vi "tkrsa6100 Config Spectrum Settings.vi"(0 "VISA Resource Name":refnum<visa-resource-name>, 1 "Set/Read\nSpectrum Setting (SET)":enum16{"SET", "READ"}(ring), 2 "Spectrum Settings\n (CENTER FREQUENCY)":T2(ring), 3 "Center Freq\n(MHz)(100)":dbl=100.0 min=0.0 max=20000.0 step=1e-06, 4 "Freq Span\n(MHz)(40)":dbl=40.0 min=1e-05 max=20000.0 step=1e-06, 5 "error in (no error)":errorcluster, 6 "Start Freq\n(MHz)(100)":dbl=100.0 min=0.0 max=14000.0 step=1e-06, 7 "Stop Freq\n(MHz)(1000)":dbl=1000.0 min=0.0 max=14000.0 step=1e-06, 8 "Freq Step\n(MHz)(10)":dbl=10.0 min=0.0 max=14000.0 step=1e-06, 9 "# Points\n(801)":enum16{"801", "2401", "4001", "8001", "10401"}(ring), 10 "Optimization\n(AUTO)":enum16{"AUTO", "DYNAMIC RANGE", "MIN NOISE"}(ring), 11 "Res BW (KHz)\n(300)":dbl=300.0 min=0.001 max=10000.0 step=0.001 format="%#_6f", 12 "Window\n(UNIFORM)":T1(ring)) -> (14 "dup VISA Resource Name":refnum<visa-resource-name>, 15 "Spectrum Setting\nResponse String":string, 19 "error out":errorcluster {"code" format="%#.0f"})   [LabVIEW 2020, in "Library Instrument & Equipement.lvlib" / "Library Spectrum Analyser.lvlib"]
doc: "Prerequisites for use:\n \nThis VI is valid in the Spectrum measurement view available in the General Signal Viewing measurement group.\n\nThis VI controls the following spectrum analysis functions:\nSets/reads center frequency\nSets/reads frequency span\nSets analyzer directly to maximum real-time span\nSets/reads resolution bandwidth\nSets/reads start frequency\nSets/reads stop frequency\nSets/reads frequency step size\nSets/reads state of auto frequency step function\nSets/reads state of auto resolution function\nSets/reads FFT window type\nSets/reads # of spectrum points\nSets/reads whether the analyzer is using resolution bandwidth or FFT windowing\nSets/reads the type of gain/bandwidth optimization in use\n\nerror in (no error) is checked by tkrsa6100 Write/Read wError Query.vi for any pending errors.\n\nIf error in status is ERROR:\n\nerror in (no error) and VISA Resource Name are passed straight through to error out and dup VISA Resource Name of the Write/Read Drivers and returned to the calling function. No commands are processed.\n\nIf error in status is NO ERROR:\n\nBy passing SET to Set/Read Spectrum Settings (SET) the following parameters can be written. Pass the following functions to Spectrum Settings (CENTER FREQUENCY). Additional parameters to be passed are specified with each function.\n\nOne command/query is executed per VI call.\n\nCENTER FREQUENCY \nSets the center frequency of the spectrum analyzer. Pass the desired frequency in MHz to numeric control Center Freq (MHz)(100).\n\nFREQUENCY SPAN\nSets the frequency span of the spectrum analyzer. Pass the desired span in MHz to numeric control Freq Span (MHz)(40).\n\nRESOLUTION BANDWIDTH\nSets the resolution bandwidth of the spectrum analyzer. Pass the desired bandwidth in KHz to numeric control Res BW (KHz)(300).\n\nMAX REAL TIME SPAN (SET)\nSet Only\nSets the frequency span of the spectrum analyzer to its maximum real time available value. No further parameters necessary to be passed.\n\nSTART FREQUENCY\nSets the start frequency of the spectrum analyzer. Pass the desired frequency in MHz to numeric control Start Freq (MHz)(100).\n\nSTOP FREQUENCY\nSets the stop frequency of the spectrum analyzer. Pass the desired frequency in MHz to numeric control Stop Freq (MHz)(100).\n\nFREQ STEP SIZE\nSets the step size for incrementing/decrementing center frequency of the spectrum analyzer in MHz. Pass the desired step in MHz to numeric control Freq Step (MHz)(2).\n\nAUTO FREQ STEP ON\nAUTO FREQ STEP OFF\nEnables/disables the spectrum analyzer's auto frequency step function. No further parameters necessary to be passed.\n\nAUTO RES BW ON\nAUTO RES BW OFF\nEnables/disables the spectrum analyzer's auto resolution bandwidth function. No further parameters necessary to be passed.\n\nFFT WINDOW TYPE\nSelects the FFT window type to use when the bandwidth method is set to FFT with the RBW Process Off function included in this driver. Pass the desired window type to enumerated control Window (UNIFORM).\n\nNote: If this function is used when RBW Process On has been selected, error -200 \"Can't set the window when in RBW mode\" is returned.\n\nRBW PROCESS ON\nRBW PROCESS OFF\nSets the bandwidth mode of the spectrum analyzer to Resolution Bandwidth (On) or FFT Window (Off). No further parameters necessary to be passed.\n\nGAIN/BW OPTIMIZATION\nSets the desired result of the gain/bandwidth optimization function of the spectrum analyzer. Pass the desired value to enumerated control Optimization (AUTO).\n\nThe following parameters can be read by passing READ to enumerated control Set/Read Spectrum Settings (SET). Pass the following values to Spectrum Settings (CENTER FREQUENCY). The current values are returned in string indicator Spectrum Settings Response String.\n\nCENTER FREQUENCY \nReads the current center frequency of the spectrum analyzer in Hz. No further parameters necessary to be passed.\n\nValid Return Value Range:\n\n0 to 6.2e9 (RSA6106A)\n0 to 14e9 (RSA6114A)\n\nFREQUENCY SPAN\nReads the current frequency span of the spectrum analyzer in Hz. No further parameters necessary to be passed.\n\nValid Return Value Range:\n\n0 to 6.2e9 (RSA6106A)\n0 to 14e9 (RSA6114A)\n\nRESOLUTION BANDWIDTH\nReads the current resolution bandwidth of the spectrum analyzer in Hz. No further parameters necessary to be passed.\n\nValid Return Value Range: 1 to 10e6\n\nSTART FREQUENCY\nReads the current start frequency of the spectrum analyzer in Hz. No further parameters necessary to be passed.\n\nValid Return Value Range:\n\n0 to 6.2e9 (RSA6106A)\n0 to 14e9 (RSA6114A)\n\nSTOP FREQUENCY\nReads the current stop frequency of the spectrum analyzer in Hz. No further parameters necessary to be passed.\n\nValid Return Value Range:\n\n0 to 6.2e9 (RSA6106A)\n0 to 14e9 (RSA6114A)\n\nFREQ STEP SIZE\nReads the current frequency step size for incrementing/decrementing center frequency of the spectrum analyzer in Hz. No further parameters necessary to be passed.\n\nValid Return Value Range:\n\n0 to 6.2e9 (RSA6106A)\n0 to 14e9 (RSA6114A)\n\nAUTO FREQ STEP ON\nAUTO FREQ STEP OFF\nEither selection reads the current state of the spectrum analyzer's auto frequency step function. No further parameters necessary to be passed.\n\nValid Return Values:\n\n0 (Off)\n1 (On)\n\nAUTO RES BW ON\nAUTO RES BW OFF\nEither selection reads the current state of the spectrum analyzer's auto resolution bandwidth function. No further parameters necessary to be passed.\n\nValid Return Values:\n\n0 (Off)\n1 (On)\n\nFFT WINDOW TYPE\nReads the FFT window type currently in use. No further parameters necessary to be passed.\n\nValid Return Values:\n\nUNIF (Uniform)\nBH4B (Blackman Harris 4B)\nFLAT (Flattop)\nHANN (Hanning)\nKAIS (Kaiser)\n\nRBW PROCESS ON\nRBW PROCESS OFF\nEither selection reads whether the analyzer is set to use resolution bandwidth processing or FFT windowing. No further parameters necessary to be passed.\n\nValid Return Values:\n\n0 (FFT)\n1 (Resolution BW)\n\nGAIN/BW OPTIMIZATION\nReads the current setting of the gain/bandwidth optimization function of the spectrum analyzer. No further parameters necessary to be passed.\n\nValid Return Values:\n\nAUTO (Auto)\nMAXD (Max Dynamic Range)\nMINN (Minimum Noise)\n\nThe appropriate command/query string is passed to tkrsa6100 Write/Read wError Query.vi. VI Input Error Query? is set to YES so query SYST:ERR? is appended to the command string and any current error information is displayed in cluster Error Out. \nOn completion dup VISA Resource Name, Error Out, and Spectrum Settings Response String are returned to the calling function."
uses:
  Library Spectrum Analyser.lvlib
panel:
  # "RSA6100 Config Spectrum Settings Driver"
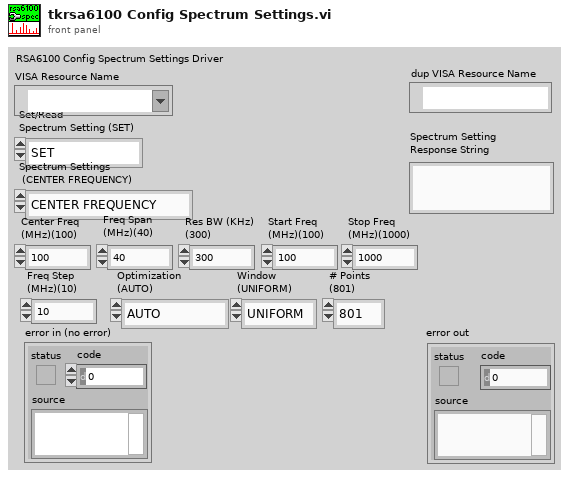
[diagram p1: front panel]
types:
  T1 = enum16{"UNIFORM", "BH4B", "FLATTOP", "HANNING", "KAISER"}
  T2 = enum16{"CENTER FREQUENCY", "FREQUENCY SPAN", "RESOLUTION BW", "MAX REAL TIME SPAN (SET)", "START FREQUENCY", "STOP FREQUENCY", "FREQ STEP SIZE", "AUTO FREQ STEP ON", "AUTO FREQ STEP OFF", "AUTO RES BW ON", "AUTO RES BW OFF", "FFT WINDOW TYPE", "# POINTS", "RBW PROCESS ON", "RBW PROCESS OFF", "GAIN/BW OPTIMIZATION"}
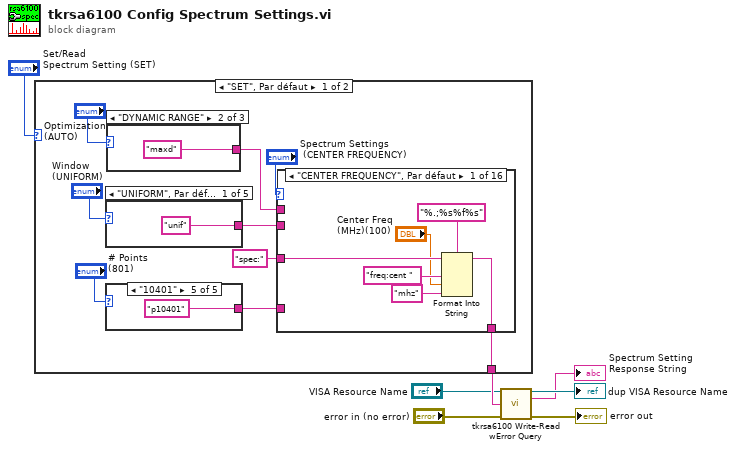
[diagram p0: block diagram]
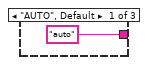
[diagram p2: hidden frame]
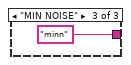
[diagram p3: hidden frame]
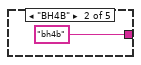
[diagram p4: hidden frame]
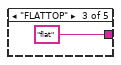
[diagram p5: hidden frame]
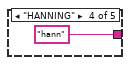
[diagram p6: hidden frame]
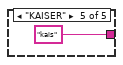
[diagram p7: hidden frame]
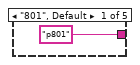
[diagram p8: hidden frame]
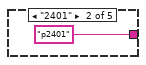
[diagram p9: hidden frame]
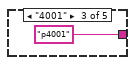
[diagram p10: hidden frame]
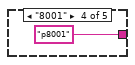
[diagram p11: hidden frame]
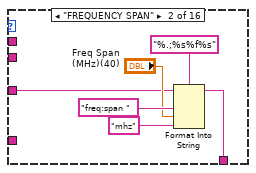
[diagram p12: hidden frame]
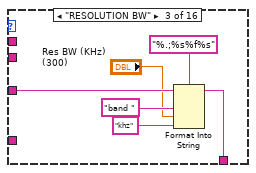
[diagram p13: hidden frame]
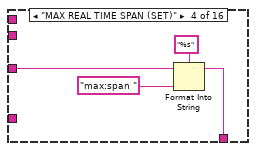
[diagram p14: hidden frame]
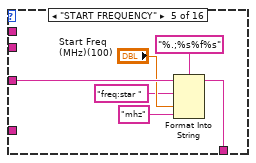
[diagram p15: hidden frame]
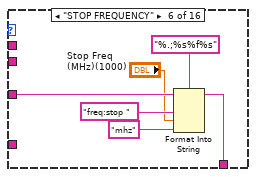
[diagram p16: hidden frame]
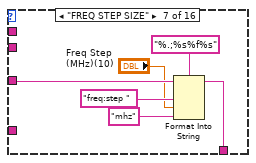
[diagram p17: hidden frame]
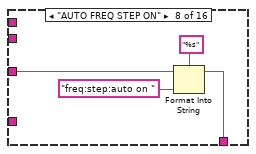
[diagram p18: hidden frame]
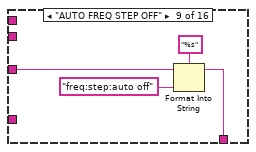
[diagram p19: hidden frame]
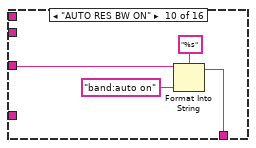
[diagram p20: hidden frame]
diagram:
  n1 = case shown="\"SET\", Par défaut" "Set/Read\nSpectrum Setting (SET)" {
    tunnel: [w16 w110] -> w3
    frame "SET", Default {
      n2 = case shown="\"UNIFORM\", Par défaut" "Window\n(UNIFORM)" {
        tunnel: ["unif" ("initial string") "bh4b" ("initial string") "flat" ("initial string") "hann" ("initial string") "kais" ("initial string")] -> w9
        frame "UNIFORM", Default {
        }
        frame "BH4B" {
        }
        frame "FLATTOP" {
        }
        frame "HANNING" {
        }
        frame "KAISER" {
        }
      }
      n3 = case shown="\"10401\"" "# Points\n(801)" {
        tunnel: ["p801" ("initial string") "p2401" ("initial string") "p4001" ("initial string") "p8001" ("initial string") "p10401" ("initial string")] -> w12
        frame "801", Default {
        }
        frame "2401" {
        }
        frame "4001" {
        }
        frame "8001" {
        }
        frame "10401" {
        }
      }
      n4 = case shown="\"DYNAMIC RANGE\"" "Optimization\n(AUTO)" {
        tunnel: ["auto" ("initial string") "maxd" ("initial string") "minn" ("initial string")] -> w8
        frame "AUTO", Default {
        }
        frame "DYNAMIC RANGE" {
        }
        frame "MIN NOISE" {
        }
      }
      n5 = case shown="\"CENTER FREQUENCY\", Par défaut" "Spectrum Settings\n (CENTER FREQUENCY)" {
        tunnel: [w34 w40 w46 w50 w56 w62 w68 w72 w76 w80 w84 w89 w94 w98 w102 w107] -> w16
        tunnel: "spec:" ("initial string") -> [w31 w36 w43 w48 w54 w59 w65 w70 w74 w78 w82 w87 w92 w96 w100 w105]
        tunnel: w12 -> [_ _ _ _ _ _ _ _ _ _ _ _ w91 _ _ _]
        tunnel: w9 -> [_ _ _ _ _ _ _ _ _ _ _ w86 _ _ _ _]
        tunnel: w8 -> [_ _ _ _ _ _ _ _ _ _ _ _ _ _ _ w104]
        frame "CENTER FREQUENCY", Default {
          n6 = Format Into String(format string="%.;%s%f%s", initial string=w31, "freq:cent " ("initial string"), "Center Freq\n(MHz)(100)", "mhz" ("input 2")) -> (resulting string=w34:string)  [unwired: 1 in, 1 out]
        }
        frame "FREQUENCY SPAN" {
          n7 = Format Into String(format string="%.;%s%f%s", initial string=w36, "freq:span " ("initial string"), "Freq Span\n(MHz)(40)", "mhz" ("input 2")) -> (resulting string=w40:string)  [unwired: 1 in, 1 out]
        }
        frame "RESOLUTION BW" {
          n8 = Format Into String(format string="%.;%s%f%s", initial string=w43, "band " ("initial string"), "Res BW (KHz)\n(300)", "khz" ("input 2")) -> (resulting string=w46:string)  [unwired: 1 in, 1 out]
        }
        frame "MAX REAL TIME SPAN (SET)" {
          n9 = Format Into String(format string="%s", initial string=w48, "max:span " ("initial string")) -> (resulting string=w50:string)  [unwired: 1 in, 1 out]
        }
        frame "START FREQUENCY" {
          n10 = Format Into String(format string="%.;%s%f%s", initial string=w54, "freq:star " ("input 1"), "Start Freq\n(MHz)(100)", "mhz" ("input 2")) -> (resulting string=w56:string)  [unwired: 1 in, 1 out]
        }
        frame "STOP FREQUENCY" {
          n11 = Format Into String(format string="%.;%s%f%s", initial string=w59, "freq:stop " ("initial string"), "Stop Freq\n(MHz)(1000)", "mhz" ("input 2")) -> (resulting string=w62:string)  [unwired: 1 in, 1 out]
        }
        frame "FREQ STEP SIZE" {
          n12 = Format Into String(format string="%.;%s%f%s", initial string=w65, "freq:step " ("initial string"), "Freq Step\n(MHz)(10)", "mhz" ("input 2")) -> (resulting string=w68:string)  [unwired: 1 in, 1 out]
        }
        frame "AUTO FREQ STEP ON" {
          n13 = Format Into String(format string="%s", initial string=w70, "freq:step:auto on " ("initial string")) -> (resulting string=w72:string)  [unwired: 1 in, 1 out]
        }
        frame "AUTO FREQ STEP OFF" {
          n14 = Format Into String(format string="%s", initial string=w74, "freq:step:auto off" ("initial string")) -> (resulting string=w76:string)  [unwired: 1 in, 1 out]
        }
        frame "AUTO RES BW ON" {
          n15 = Format Into String(format string="%s", initial string=w78, "band:auto on" ("initial string")) -> (resulting string=w80:string)  [unwired: 1 in, 1 out]
        }
        frame "AUTO RES BW OFF" {
          n16 = Format Into String(format string="%s", initial string=w82, "band:auto off" ("initial string")) -> (resulting string=w84:string)  [unwired: 1 in, 1 out]
        }
        frame "FFT WINDOW TYPE" {
          n17 = Format Into String(format string="%s%s", initial string=w87, "fft:wind " ("initial string"), w86) -> (resulting string=w89:string)  [unwired: 1 in, 1 out]
        }
        frame "# POINTS" {
          n18 = Format Into String(format string="%s%s", initial string=w92, "poin:coun " ("initial string"), w91) -> (resulting string=w94:string)  [unwired: 1 in, 1 out]
        }
        frame "RBW PROCESS ON" {
          n19 = Format Into String(format string="%s", initial string=w96, "band:mode on" ("initial string")) -> (resulting string=w98:string)  [unwired: 1 in, 1 out]
        }
        frame "RBW PROCESS OFF" {
          n20 = Format Into String(format string="%s", initial string=w100, "band:mode off" ("initial string")) -> (resulting string=w102:string)  [unwired: 1 in, 1 out]
        }
        frame "GAIN/BW OPTIMIZATION" {
          n21 = Format Into String(format string="%s%s", initial string=w105, "band:opt " ("initial string"), w104) -> (resulting string=w107:string)  [unwired: 1 in, 1 out]
        }
      }
    }
    frame "READ" {
      n22 = local read "Spectrum Settings\n (CENTER FREQUENCY)"() -> (w111:T2)
      n23 = case shown="\"STOP FREQUENCY\"" w111 {
        tunnel: [w112 w116 w120 w124 w128 w132 w136 w140 w144 w148 w152 w156 w160 w164 w168 w172] -> w110
        tunnel: "spec:" -> [w114 w118 w122 w126 w130 w134 w138 w142 w146 w150 w154 w158 w162 w166 w170 w174]
        frame "CENTER FREQUENCY", Default {
          n24 = Format Into String(format string="%s", initial string=w114, "freq:cent?") -> (resulting string=w112:string)  [unwired: 1 in, 1 out]
        }
        frame "FREQUENCY SPAN" {
          n25 = Format Into String(format string="%s", initial string=w118, "freq:span?") -> (resulting string=w116:string)  [unwired: 1 in, 1 out]
        }
        frame "FREQ STEP SIZE" {
          n26 = Format Into String(format string="%s", initial string=w122, "freq:step?") -> (resulting string=w120:string)  [unwired: 1 in, 1 out]
        }
        frame "AUTO FREQ STEP ON" {
          n27 = Format Into String(format string="%s", initial string=w126, "freq:step:auto?") -> (resulting string=w124:string)  [unwired: 1 in, 1 out]
        }
        frame "AUTO FREQ STEP OFF" {
          n28 = Format Into String(format string="%s", initial string=w130, "freq:step:auto?") -> (resulting string=w128:string)  [unwired: 1 in, 1 out]
        }
        frame "START FREQUENCY" {
          n29 = Format Into String(format string="%s", initial string=w134, "freq:star?") -> (resulting string=w132:string)  [unwired: 1 in, 1 out]
        }
        frame "AUTO RES BW ON" {
          n30 = Format Into String(format string="%s", initial string=w138, "band:auto?") -> (resulting string=w136:string)  [unwired: 1 in, 1 out]
        }
        frame "AUTO RES BW OFF" {
          n31 = Format Into String(format string="%s", initial string=w142, "band:auto?") -> (resulting string=w140:string)  [unwired: 1 in, 1 out]
        }
        frame "FFT WINDOW TYPE" {
          n32 = Format Into String(format string="%s", initial string=w146, "fft:wind?") -> (resulting string=w144:string)  [unwired: 1 in, 1 out]
        }
        frame "RBW PROCESS ON" {
          n33 = Format Into String(format string="%s", initial string=w150, "band:mode?") -> (resulting string=w148:string)  [unwired: 1 in, 1 out]
        }
        frame "RBW PROCESS OFF" {
          n34 = Format Into String(format string="%s", initial string=w154, "band:mode?") -> (resulting string=w152:string)  [unwired: 1 in, 1 out]
        }
        frame "GAIN/BW OPTIMIZATION" {
          n35 = Format Into String(format string="%s", initial string=w158, "band:opt?") -> (resulting string=w156:string)  [unwired: 1 in, 1 out]
        }
        frame "RESOLUTION BW" {
          n36 = Format Into String(format string="%s", initial string=w162, "band?") -> (resulting string=w160:string)  [unwired: 1 in, 1 out]
        }
        frame "MAX REAL TIME SPAN (SET)" {
          n37 = Format Into String(format string="%s", initial string=w166, "max:span?") -> (resulting string=w164:string)  [unwired: 1 in, 1 out]
        }
        frame "STOP FREQUENCY" {
          n38 = Format Into String(format string="%s", initial string=w170, "freq:stop?") -> (resulting string=w168:string)  [unwired: 1 in, 1 out]
        }
        frame "# POINTS" {
          n39 = Format Into String(format string="%s", initial string=w174, "poin:coun?") -> (resulting string=w172:string)  [unwired: 1 in, 1 out]
        }
      }
    }
  }
  n40 = call "tkrsa6100 Write-Read wError Query.vi"("VISA Resource Name"="VISA Resource Name", "Command (Empty String)"=w3, "error in (no error)"="error in (no error)") -> ("dup VISA Resource Name"=→"dup VISA Resource Name":refnum<visa-resource-name>, "Response"=→"Spectrum Setting\nResponse String":string, "error out"=→"error out":errorcluster)  [unwired: 4 in, 6 out]
